vi "tm_setemprotection_40.vi"(8 "error in (no error)":errorcluster, 10 "Parameters":T1={"Mode"=FALSE, "Alarm"=FALSE, "Level"=1, "Frames"=0} {"Level" min=1 max=3 step=1}, 11 "Handle in":u32) -> (0 "error out":errorcluster, 3 "Handle out":u32)   [LabVIEW 2023]
uses:
  tmcamcon.dll
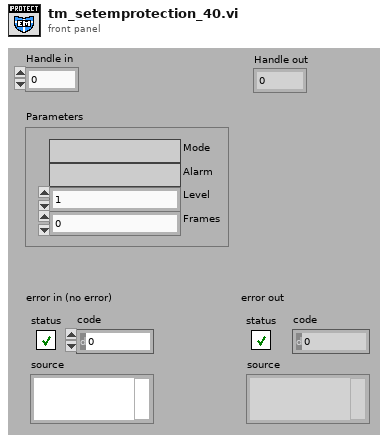
[diagram p1: front panel]
types:
  T1 = cluster{"Mode":bool, "Alarm":bool, "Level":i32, "Frames":i32}
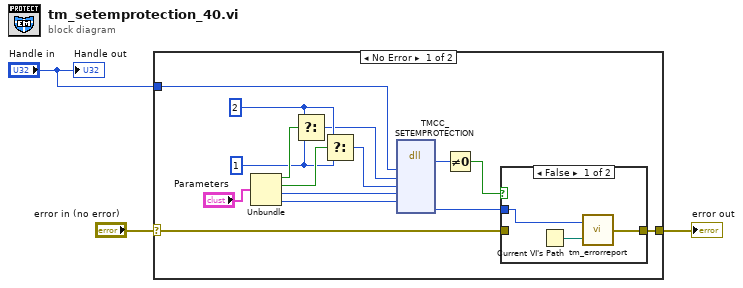
[diagram p0: block diagram]
diagram:
  n1 = case shown="No Error" "error in (no error)" {
    selector: "error in (no error)" -> [w13 w23]
    tunnel: [w10 w23] -> w2
    tunnel: "Handle in" -> [w14 _]
    frame No Error {
      w7 = 2
      w6 = 1
      n2 = Unbundle("Parameters") -> ("Mode"=w9:bool, "Alarm"=w8:bool, "Level"=w16:i32, "Frames"=w15:i32)
      n3 = Select(t=w7, s=w9, f=w6) -> (s? t:f=w5:i32)
      n4 = Select(t=w7, s=w8, f=w6) -> (s? t:f=w4:i32)
      n5 = dll-call lib="tmcamcon.dll" fn="TMCC_SETEMPROTECTION"("HDCAM"=w14, "mode"=w5, "alarm"=w4, "level"=w16, "frames"=w15) -> ("return type"=w18:u32, "Erval"=w12:i32)  [unwired: 9 in, 2 out]
      n6 = Not Equal To 0?(x=w18) -> (x != 0?=w11:bool)
      n7 = case shown="False" w11 {
        tunnel: w13 -> [_ w22]
        tunnel: [w20 w22] -> w10
        tunnel: w12 -> [w19 _]
        frame False {
          n8 = Current VI's Path() -> (path=w21:path)
          n9 = call "tm_errorreport.vi"("Source"=w21, "Error"=w19) -> ("error out"=w20:errorcluster)
        }
        frame True {
        }
      }
    }
    frame Error {
    }
  }
  "error out" <- w2
  "Handle out" <- "Handle in"
